vi "move_.vi"(0 "Enum":enum16{"hold", "f", "b"}(ring), 2 "delay":u32, 3 "D":dbl) -> ()   [LabVIEW 2017]
uses:
  GlobalVar.vi
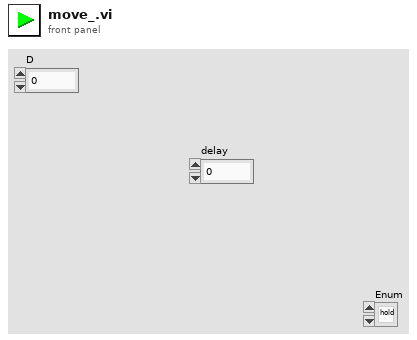
[diagram p1: front panel]
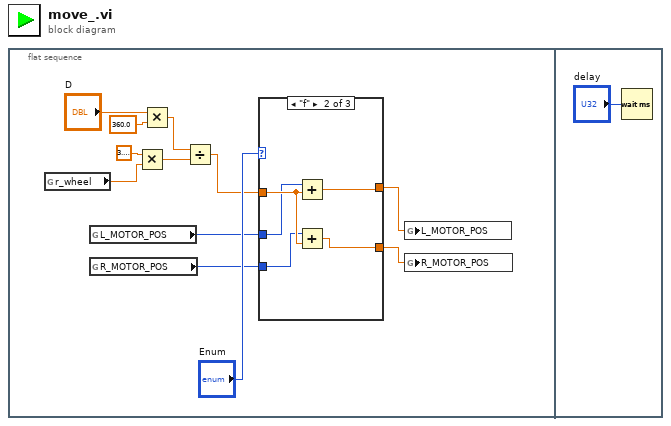
[diagram p0: block diagram]
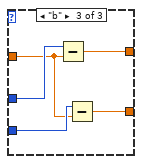
[diagram p3: hidden frame]
diagram:
  n1 = flat-sequence {
    frame #0 {
      n2 = global read "GlobalVar.vi" "r_wheel"() -> (w1:dbl)
      n3 = global read "GlobalVar.vi" "L_MOTOR_POS"() -> (w6:i32)
      n4 = global read "GlobalVar.vi" "R_MOTOR_POS"() -> (w5:i32)
      n5 = Multiply(x=3.141592653589793, y=w1) -> (x*y=w8:dbl)
      n6 = Multiply(x="D", y=360.0) -> (x*y=w9:dbl)
      n7 = Divide(x=w9, y=w8) -> (x/y=w4:dbl)
      n8 = case shown="\"f\"" "Enum" {
        tunnel: w6 -> [w14 w18 w24]
        tunnel: w5 -> [w13 w17 w23]
        tunnel: w4 -> [_ w19 w22]
        tunnel: [w14 w15 w21] -> w3
        tunnel: [w13 w16 w20] -> w2
        frame "hold", Default {
        }
        frame "f" {
          n9 = Add(x=w18, y=w19) -> (x+y=w15:dbl)
          n10 = Add(x=w17, y=w19) -> (x+y=w16:dbl)
        }
        frame "b" {
          n11 = Subtract(x=w24, y=w22) -> (x-y=w21:dbl)
          n12 = Subtract(x=w23, y=w22) -> (x-y=w20:dbl)
        }
      }
      n13 = global write "GlobalVar.vi" "L_MOTOR_POS"(w3) -> ()
      n14 = global write "GlobalVar.vi" "R_MOTOR_POS"(w2) -> ()
    }
    frame #1 {
      n15 = Wait (ms)(milliseconds to wait="delay") -> ()  [unwired: 1 out]
    }
  }
